vi "testDDS.vi"() -> ()   [LabVIEW 2009, in "run.lvlib"]
uses:
  testing/run.lvlib
  Generic/DDSOutput.lvclass
panel:
  out "status array":bool[](array[boolean])
  in  "Ring":u16(ring) items=["Simulated", "SpinCoreDDS0", "SpinCoreDDS1"]
  in  "stop":bool
  in  "Phase":dbl[](array[numeric])=[0.0, 0.0, 0.0]
  in  "Amp":dbl[](array[numeric])=[1.0, 1.0, 0.0]
  in  "freq":dbl[](array[numeric])=[100.0, 90.0, 100.0]
  in  "Times":dbl[](array[numeric])=[0.0, 1.0, 2.0]
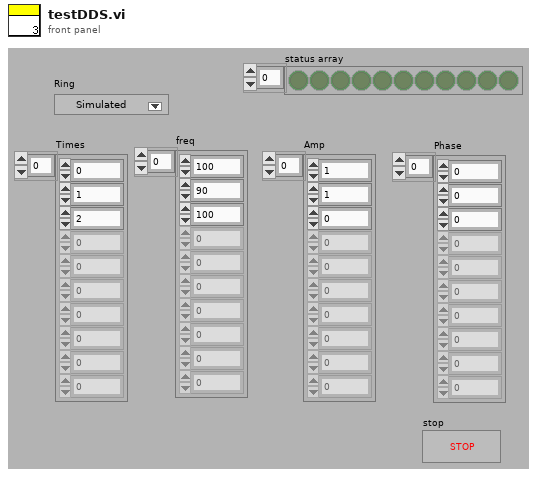
[diagram p1: front panel]
types:
  T1 = cluster{"Frequency(MHz)":dbl, "Amplitude":dbl, "Phase":dbl, "OutputForm":enum16{"Sine", "Square", "Triangle", "Arbitrary"}}[]
  T2 = cluster{"OutputForm":enum16{"Sine", "Square", "Triangle", "Arbitrary"}[], "OutputFunction":enum16{"Frequency", "Ramp", "Sequence"}[], "physicalChannels":string}
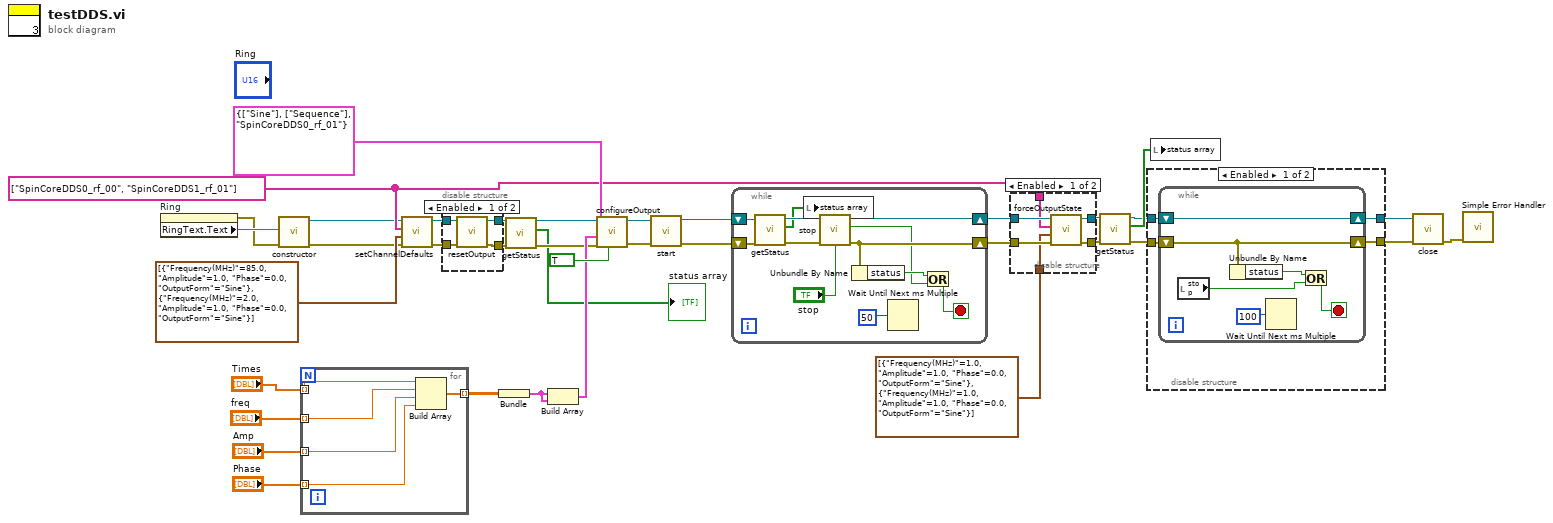
[diagram p0: block diagram]
diagram:
  w3 = string[] ["SpinCoreDDS0_rf_00", "SpinCoreDDS1_rf_01"]
  n1 = property on="Ring" class="Ring (strict)"() -> (error out=w27:errorcluster, "RingText.Text"=w28:string)  [unwired: 2 in, 1 out]
  n2 = call "constructor.vi"("error in (no error)"=w27, "device"=w28) -> ("error out"=w1:errorcluster, "DDSOutput out"=w2:refnum<class "DDSOutput.lvclass">)  [unwired: 8 in]
  n3 = for {
    tunnel: "Times" -> [w42] mode=indexing
    tunnel: "freq" -> [w41] mode=indexing
    tunnel: "Amp" -> [w40] mode=indexing
    tunnel: "Phase" -> [w39] mode=indexing
    tunnel: [w38] -> w31 mode=indexing
    n4 = Build Array(w42, w41, w40, w39) -> (w38:dbl[])
  }
  n5 = call-dynamic "setChannelDefaults.vi"("error in (no error)"=w1, "Data"=T1 [{"Frequency(MHz)"=85.0, "Amplitude"=1.0, "Phase"=0.0, "OutputForm"=enum."Sine"}, {"Frequency(MHz)"=2.0, "Amplitude"=1.0, "Phase"=0.0, "OutputForm"=enum."Sine"}] ("Defaults"), "physicalChannels"=w3, "DDSOutput in"=w2) -> ("error out"=w22:errorcluster, "DDSOutput out"=w23:refnum<class "DDSOutput.lvclass">)  [unwired: 6 in]
  n6 = disable-structure shown="Enabled" {
    disable-tunnel: w23 -> [w46 w48]
    disable-tunnel: w22 -> [w45 w47]
    disable-tunnel: [w44 w48] -> w16
    disable-tunnel: [w43 w47] -> w15
    frame #0 {
      n7 = call-dynamic "resetOutput.vi"("error in (no error)"=w45, "DDSOutput in"=w46) -> ("error out"=w43:errorcluster, "DDSOutput out"=w44:refnum<class "DDSOutput.lvclass">)  [unwired: 8 in]
    }
    frame #1 {
    }
  }
  n8 = Bundle(w31) -> (w4:cluster{dbl[][]})  [unwired: 1 in]
  n9 = call-dynamic "getStatus.vi"("error in (no error)"=w15, "DDSOutput in"=w16) -> ("error out"=w14:errorcluster, "status array"=→"status array":bool[], "DDSOutput out"=w13:refnum<class "DDSOutput.lvclass">)  [unwired: 7 in]
  n10 = Build Array(w4, w4) -> (w25:cluster{dbl[][]}[])
  n11 = call-dynamic "configureOutput.vi"("sofwareTrigger?"=TRUE, "error in (no error)"=w14, "Data"=w25, "Config"=T2 {"OutputForm"=[enum."Sine"], "OutputFunction"=[enum."Sequence"], "physicalChannels"="SpinCoreDDS0_rf_01"}, "DDSOutput in"=w13) -> ("error out"=w29:errorcluster, "DDSOutput out"=w30:refnum<class "DDSOutput.lvclass">)  [unwired: 5 in]
  n12 = call-dynamic "start.vi"("error in (no error)"=w29, "DDSOutput in"=w30) -> ("error out"=w5:errorcluster, "DDSOutput out"=w6:refnum<class "DDSOutput.lvclass">)  [unwired: 8 in]
  n13 = while {
    shift-right: [w59] -> w21
    shift-left: w6 -> [w53]
    shift-right: [w58] -> w20
    shift-left: w5 -> [w50]
    stop <- w55 stop-if-true
    n14 = call-dynamic "getStatus.vi"("error in (no error)"=w50, "DDSOutput in"=w53) -> ("error out"=w51:errorcluster, "status array"=w49:bool[], "DDSOutput out"=w52:refnum<class "DDSOutput.lvclass">)  [unwired: 7 in]
    n15 = local write "status array"(w49) -> ()
    n16 = call-dynamic "stop.vi"("error in (no error)"=w51, "stop?"="stop", "DDSOutput in"=w52) -> ("error out"=w58:errorcluster, "hasStopped"=w56:bool, "DDSOutput out"=w59:refnum<class "DDSOutput.lvclass">)  [unwired: 6 in]
    n17 = Unbundle By Name(w58) -> ("status"=w57:bool)
    n18 = Wait Until Next ms Multiple(millisecond multiple=50) -> ()  [unwired: 1 out]
    n19 = Or(x=w57, y=w56) -> (x .or. y?=w55:bool)
  }
  n20 = disable-structure shown="Enabled" {
    disable-tunnel: w21 -> [w66 w68]
    disable-tunnel: w20 -> [w65 w67]
    disable-tunnel: w3 -> [w61 _]
    disable-tunnel: T1 [{"Frequency(MHz)"=1.0, "Amplitude"=1.0, "Phase"=0.0, "OutputForm"=enum."Sine"}, {"Frequency(MHz)"=1.0, "Amplitude"=1.0, "Phase"=0.0, "OutputForm"=enum."Sine"}] ("Defaults") -> [w64 _]
    disable-tunnel: [w63 w68] -> w11
    disable-tunnel: [w62 w67] -> w10
    frame #0 {
      n21 = call-dynamic "forceOutputState.vi"("error in (no error)"=w65, "data"=w64, "physicalChannels"=w61, "DDSOutput in"=w66) -> ("error out"=w62:errorcluster, "DDSOutput out"=w63:refnum<class "DDSOutput.lvclass">)  [unwired: 6 in]
    }
    frame #1 {
    }
  }
  n22 = call-dynamic "getStatus.vi"("error in (no error)"=w10, "DDSOutput in"=w11) -> ("error out"=w7:errorcluster, "status array"=w9:bool[], "DDSOutput out"=w8:refnum<class "DDSOutput.lvclass">)  [unwired: 7 in]
  n23 = disable-structure shown="Enabled" {
    disable-tunnel: [w72 w80] -> w18
    disable-tunnel: [w71 w79] -> w17
    disable-tunnel: w8 -> [w70 w80]
    disable-tunnel: w7 -> [w69 w79]
    frame #0 {
      n24 = while {
        shift-right: [w75] -> w72
        shift-left: w70 -> [w75]
        shift-right: [w74] -> w71
        shift-left: w69 -> [w74]
        stop <- w77 stop-if-true
        n25 = local read "stop"() -> (w73:bool)
        n26 = Unbundle By Name(w74) -> ("status"=w78:bool)
        n27 = Wait Until Next ms Multiple(millisecond multiple=100) -> ()  [unwired: 1 out]
        n28 = Or(x=w78, y=w73) -> (x .or. y?=w77:bool)
      }
    }
    frame #1 {
    }
  }
  n29 = local write "status array"(w9) -> ()
  n30 = call-dynamic "close.vi"("error in (no error)"=w17, "DDSOutput in"=w18) -> ("error out"=w26:errorcluster)  [unwired: 9 in]
  n31 = call <vilib>:"Simple Error Handler.vi"("error in (no error)"=w26) -> ()  [unwired: 4 in, 5 out]
